vi "Save_Time (SubVI).vi"(8 "error in (no error)":errorcluster, 10 "group name in (Untitled)":string, 11 "Refnum in":refnum<k34>) -> (0 "error out":errorcluster, 3 "Refnum out":refnum<k34>)   [LabVIEW 2024]
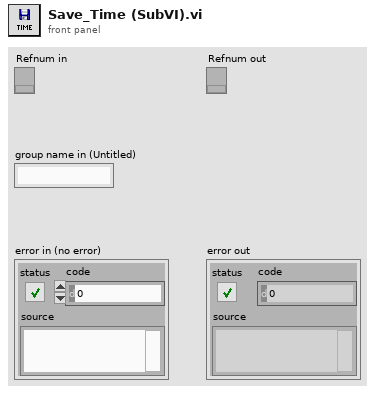
[diagram p1: front panel]
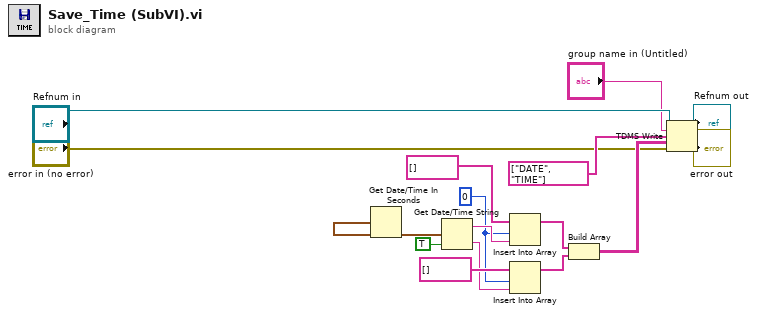
[diagram p0: block diagram]
diagram:
  w7 = 0 ("index")
  n1 = Get Date/Time In Seconds() -> (seconds since 1Jan1904=w12:timestamp)
  n2 = Get Date/Time String(seconds (now)=w12, want seconds? (F)=TRUE) -> (date string=w9:string, time string=w6:string)  [unwired: 1 in]
  n3 = Insert Into Array(array=string[] [], index=w7, new element=w9) -> (w13:string[])
  n4 = Insert Into Array(array=string[] [], index=w7, new element=w6) -> (w14:string[])
  n5 = Build Array(w13, w14) -> (w15:string[][])
  n6 = TDMS Write(0:"Refnum in", 5:"group name in (Untitled)", 7:string[] ["DATE", "TIME"], 9:w15, 11:"error in (no error)") -> (4:→"Refnum out":refnum<k34>, 15:→"error out":errorcluster)  [unwired: 1 in, 2 out]
